vi "Configure Multi Eval Meas List Segment Settings.vi"(0 "VISA resource name":refnum<visa-resource-name>, 1 "Level (0.0)":dbl format="%^.3e", 2 "Retrigger Flag (Off)":i32(ring) items=["Off", "On", "IF Power"], 5 "Instance (1)":T2=1, 7 "Segment (1)":T1=1, 9 "Segment Length (1)":i32=1, 11 "error in (no error)":errorcluster, 12 "Band (B257)":i32(ring) items=["B257", "B258", "B260", "B261"], 13 "Evaluation Offset (0)":i32) -> (4 "VISA resource name out":refnum<visa-resource-name>, 15 "error out":errorcluster)   [LabVIEW 2020, in "Rohde&Schwarz CMXP NR FR2 Measurement.lvlib"]
doc: "Defines the length and analyzer settings of segment <no>.\n\nAttribute:\nRSCMXPNRFR2M_ATTR_MULTI_EVAL_MEASUREMENT_LIST_SEGMENT_SETTINGS\n\nRemote-control command:\nCONFigure:NRMMw:MEAS<i>:LIST:SEGMent<no>:SETup"
uses:
  <instrlib>/Rohde&Schwarz CMXP NR FR2 Measurement/Rohde&Schwarz CMXP NR FR2 Measurement.lvlib
  <instrlib>/Rohde&Schwarz CMXP NR FR2 Measurement/Private/_Instance.ctl
  <instrlib>/Rohde&Schwarz CMXP NR FR2 Measurement/Private/_Segment.ctl
  <instrlib>/Rohde&Schwarz CMXP NR FR2 Measurement/Private/rsidr_core.llb/rsidr_core.lvlib
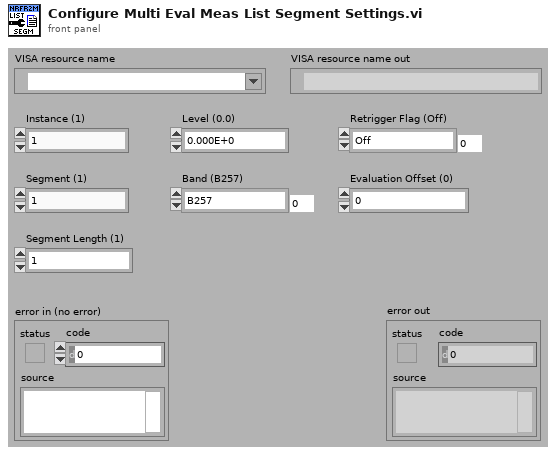
[diagram p1: front panel]
types:
  T1 = typedef "Rohde&Schwarz CMXP NR FR2 Measurement.lvlib/_Segment.ctl" = i32
  T2 = typedef "Rohde&Schwarz CMXP NR FR2 Measurement.lvlib/_Instance.ctl" = i32
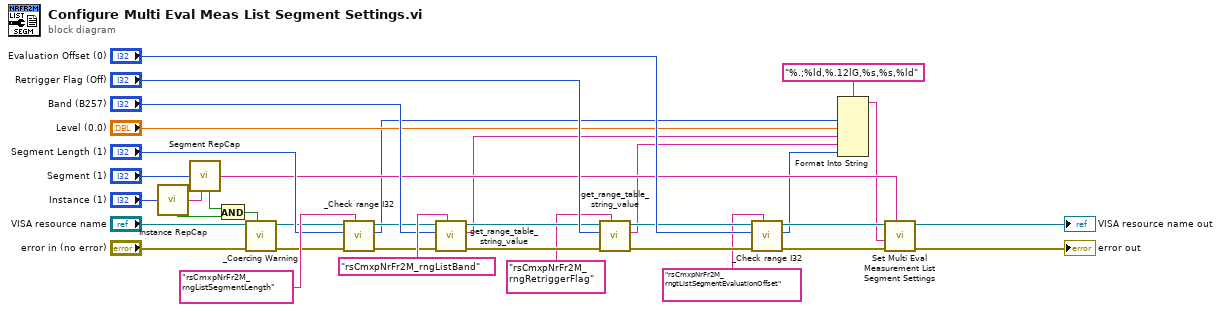
[diagram p0: block diagram]
diagram:
  n1 = call <instrlib>:"Instance RepCap.vi"("Instance In"="Instance (1)") -> ("In Range?"=w32:bool, "RepCap Identifier Out"=w4:string)  [unwired: 1 in]
  n2 = call <instrlib>:"Segment RepCap.vi"("Segment In"="Segment (1)", "RepCap String In (\"\")"=w4) -> ("In Range?"=w31:bool, "RepCap Identifier Out"=w14:string)
  n3 = And(x=w31, y=w32) -> (x .and. y?=w35:bool)
  n4 = call <instrlib>:"_Coercing Warning.vi"("In Range?"=w35, "error in (no error)"="error in (no error)", "VISA resource name"="VISA resource name") -> ("error out"=w27:errorcluster, "VISA resource name out"=w28:refnum<visa-resource-name>)  [unwired: 7 in]
  n5 = call <instrlib>:"_Check range I32.vi"("Range Table Identifier"="rsCmxpNrFr2M_rngListSegmentLength", "error in (no error)"=w27, "I32 Value In"="Segment Length (1)", "VISA resource name"=w28) -> ("error out"=w23:errorcluster, "I32 Value Out"=w9:i32, "VISA resource name out"=w24:refnum<visa-resource-name>)  [unwired: 5 in]
  n6 = call <instrlib>:"get_range_table_string_value.vi"("Range Table ID in"="rsCmxpNrFr2M_rngListBand", "error in"=w23, "I32 input"="Band (B257)", "VISA resource name"=w24) -> ("error out"=w20:errorcluster, "String Value out"=w8:string, "VISA resource name out"=w21:refnum<visa-resource-name>)  [unwired: 5 in]
  n7 = call <instrlib>:"get_range_table_string_value.vi"("Range Table ID in"="rsCmxpNrFr2M_rngRetriggerFlag", "error in"=w20, "I32 input"="Retrigger Flag (Off)", "VISA resource name"=w21) -> ("error out"=w17:errorcluster, "String Value out"=w7:string, "VISA resource name out"=w18:refnum<visa-resource-name>)  [unwired: 5 in]
  n8 = call <instrlib>:"_Check range I32.vi"("Range Table Identifier"="rsCmxpNrFr2M_rngtListSegmentEvaluationOffset", "error in (no error)"=w17, "I32 Value In"="Evaluation Offset (0)", "VISA resource name"=w18) -> ("error out"=w13:errorcluster, "I32 Value Out"=w6:i32, "VISA resource name out"=w12:refnum<visa-resource-name>)  [unwired: 5 in]
  n9 = Format Into String(format string="%.;%ld,%.12lG,%s,%s,%ld", w9, "Level (0.0)", w8, w7, w6) -> (resulting string=w3:string)  [unwired: 2 in, 1 out]
  n10 = call "Set Multi Eval Measurement List Segment Settings"("Repeated Capabilities"=w14, "error in (no error)"=w13, "Multi Eval Measurement List Segment Settings ()"=w3, "instrument handle"=w12) -> ("error out"=→"error out":errorcluster, "instrument handle out"=→"VISA resource name out":refnum<visa-resource-name>)  [unwired: 6 in]
